vi "Scan stderr.vi"(8 "error in (no error)":errorcluster, 9 "stderr in":u8[](array[numeric]), 10 "patterns":T1, 11 "client in":refnum<class "Generic Client.lvclass">) -> (0 "error out":errorcluster, 1 "stderr out":u8[](array[numeric]), 3 "client out":refnum<class "Generic Client.lvclass">)   [LabVIEW 2020, in "NI_SSH.lvlib" / "Generic Client.lvclass"]
uses:
  <vilib>/net/SSH/Client/Generic/Generic Client.lvclass
  <vilib>/net/SSH/Client/Generic/Stderr Match Patterns.ctl
  <vilib>/net/SSH/Client/Generic/Generic Client.lvclass/Generic Client.ctl
  <vilib>/net/SSH/Client/Generic/Write untrusted fingerprint.vi
  <vilib>/net/SSH/Client/Generic/Write untrusted fingerprint is incorrect_.vi
  <vilib>/Utility/error.llb/Error Cluster From Error Code.vi
  <vilib>/regexp/Match Regular Expression.xnode
  <vilib>/ErrorRing/Error Ring.xnode
  <vilib>/net/SSH/NI_SSH.lvlib
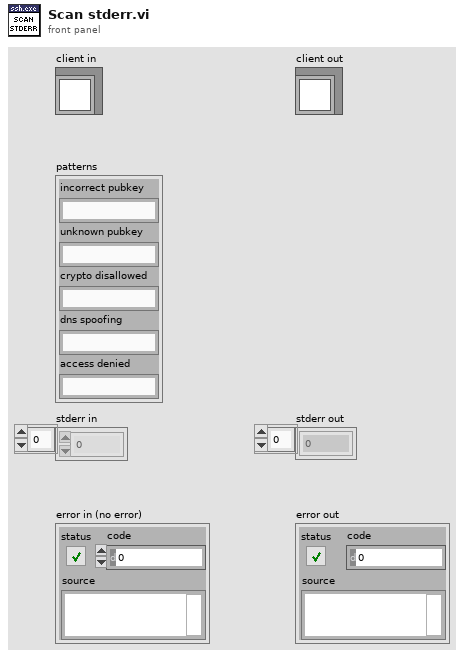
[diagram p1: front panel]
types:
  T1 = typedef "NI_SSH.lvlib/Generic Client.lvclass/Stderr Match Patterns.ctl" = cluster{"incorrect pubkey":string, "unknown pubkey":string, "crypto disallowed":string, "dns spoofing":string, "access denied":string}
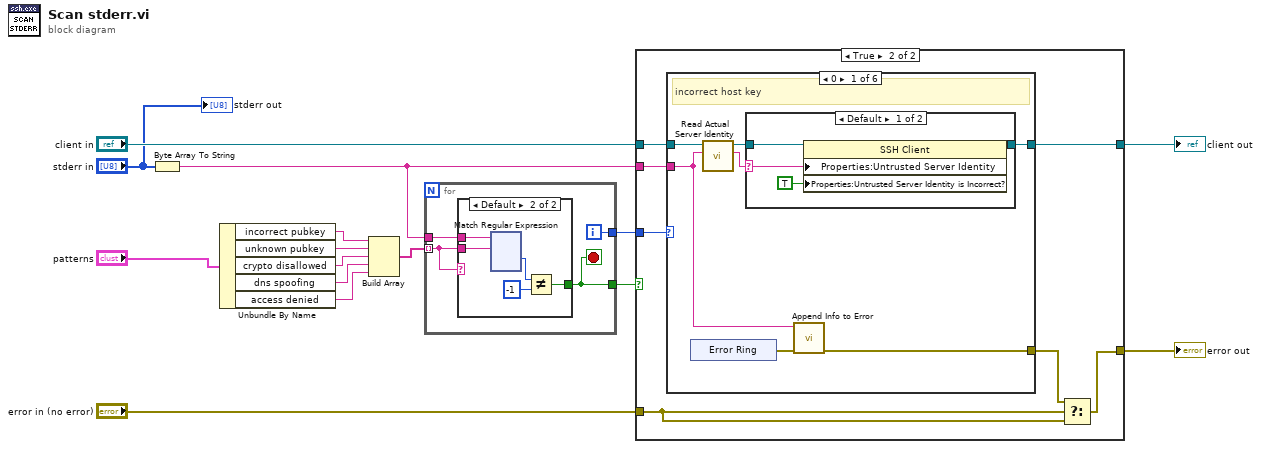
[diagram p0: block diagram]
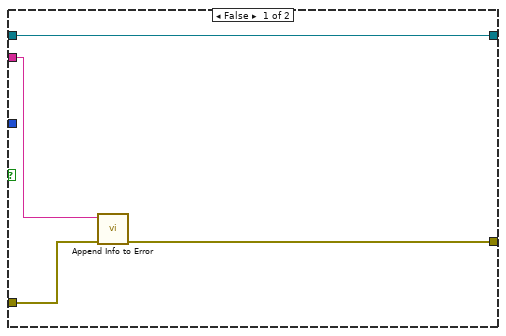
[diagram p2: hidden frame]
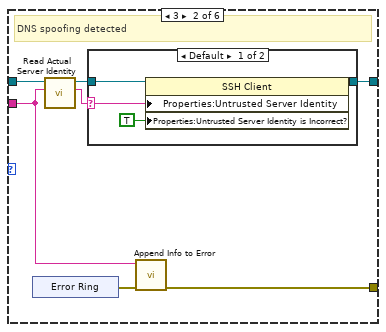
[diagram p4: hidden frame]
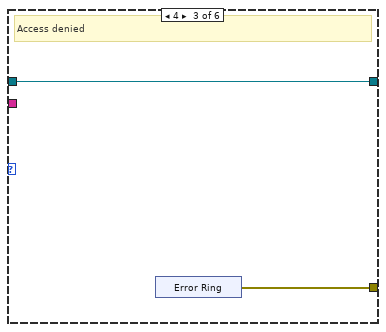
[diagram p6: hidden frame]
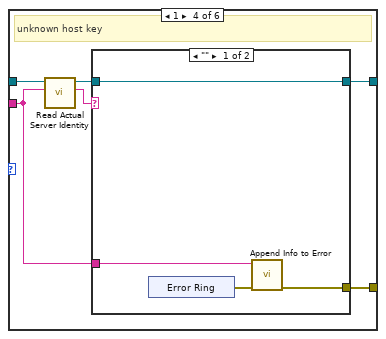
[diagram p7: hidden frame]
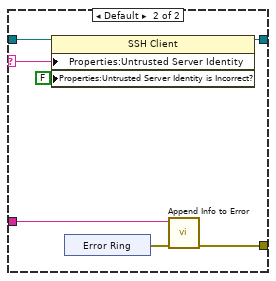
[diagram p8: hidden frame]
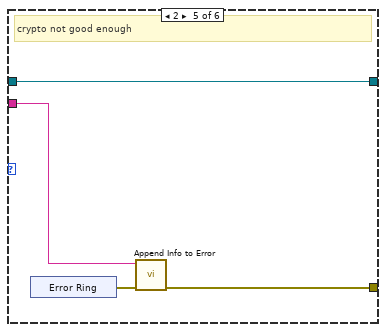
[diagram p9: hidden frame]
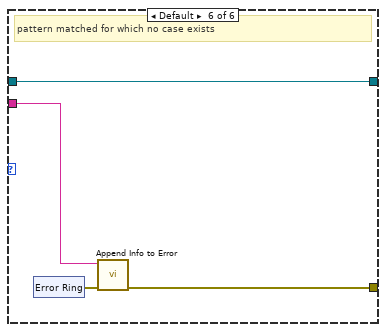
[diagram p10: hidden frame]
diagram:
  n1 = Byte Array To String(unsigned byte array="stderr in") -> (string=w12:string)
  n2 = Unbundle By Name("patterns") -> ("incorrect pubkey"=w6:string, "unknown pubkey"=w5:string, "crypto disallowed"=w4:string, "dns spoofing"=w2:string, "access denied"=w1:string)
  n3 = Build Array(w6, w5, w4, w2, w1) -> (w3:string[])
  n4 = for {
    tunnel: w12 -> [w17]
    tunnel: [w19] -> w8
    tunnel: w3 -> [w16] mode=indexing
    tunnel: [w18] -> w7
    i -> [w18]
    stop <- w19 stop-if-true
    n5 = case shown="Default" w16 {
      tunnel: [_ w23] -> w19
      tunnel: w17 -> [_ w22]
      tunnel: w16 -> [_ w21]
      frame "" {
      }
      frame Default {
        n6 = xnode ("Match Regular Expression")("input string"=w22, "regular expression"=w21) -> ("offset past match"=w20:i32)  [unwired: 4 in, 4 out]
        n7 = Not Equal?(x=w20, y=-1 ("offset past match")) -> (x != y?=w23:bool)
      }
    }
  }
  n8 = case shown="True" w8 {
    tunnel: [w140 w143] -> w11
    tunnel: "error in (no error)" -> [w141 w145]
    tunnel: w12 -> [w139 w148]
    tunnel: "client in" -> [w142 w147]
    tunnel: w7 -> [_ w149]
    tunnel: [w142 w146] -> w15
    frame False {
      n9 = call <vilib>:"Append Info to Error.vi"("error in (no error)"=w141, "additional info"=w139) -> ("error out"=w140:errorcluster)  [unwired: 9 in]
    }
    frame True {
      n10 = case shown="0" w149 {
        tunnel: [w154 w170 w182 w190 w215 w223] -> w144
        tunnel: w148 -> [w152 w168 _ w191 w213 w222]
        tunnel: w147 -> [w150 w166 w183 w188 w216 w224]
        tunnel: [w155 w171 w183 w192 w216 w224] -> w146
        frame 0 {
          # "incorrect host key"
          n11 = xnode ("Error Ring")() -> ("error out"=w153:errorcluster)
          n12 = call-dynamic "Read Actual Server Identity.vi"("server errors"=w152, "client in"=w150) -> ("fingerprint"=w156:string, "client out"=w151:refnum<class "Generic Client.lvclass">)  [unwired: 8 in]
          n13 = case shown="Default" w156 {
            selector: w156 -> [w163 _]
            tunnel: w151 -> [w164 w165]
            tunnel: [w161 w165] -> w155
            frame Default {
              n14 = property on="Property Node" class="SSH Client"(reference=w164, "Properties:Untrusted Server Identity"=w163, "Properties:Untrusted Server Identity is Incorrect?"=TRUE ("untrusted fingerprint is incorrect?")) -> (reference out=w161:refnum<class "Generic Client.lvclass">)  [unwired: 1 in, 1 out]
            }
            frame "" {
            }
          }
          n15 = call <vilib>:"Append Info to Error.vi"("error in (no error)"=w153, "additional info"=w152) -> ("error out"=w154:errorcluster)  [unwired: 9 in]
        }
        frame 3 {
          # "DNS spoofing detected"
          n16 = xnode ("Error Ring")() -> ("error out"=w169:errorcluster)
          n17 = call-dynamic "Read Actual Server Identity.vi"("server errors"=w168, "client in"=w166) -> ("fingerprint"=w172:string, "client out"=w167:refnum<class "Generic Client.lvclass">)  [unwired: 8 in]
          n18 = case shown="Default" w172 {
            selector: w172 -> [w179 _]
            tunnel: w167 -> [w180 w181]
            tunnel: [w177 w181] -> w171
            frame Default {
              n19 = property on="Property Node" class="SSH Client"(reference=w180, "Properties:Untrusted Server Identity"=w179, "Properties:Untrusted Server Identity is Incorrect?"=TRUE ("untrusted fingerprint is incorrect?")) -> (reference out=w177:refnum<class "Generic Client.lvclass">)  [unwired: 1 in, 1 out]
            }
            frame "" {
            }
          }
          n20 = call <vilib>:"Append Info to Error.vi"("error in (no error)"=w169, "additional info"=w168) -> ("error out"=w170:errorcluster)  [unwired: 9 in]
        }
        frame 4 {
          # "Access denied"
          n21 = xnode ("Error Ring")() -> ("error out"=w182:errorcluster)
        }
        frame 1 {
          # "unknown host key"
          n22 = call-dynamic "Read Actual Server Identity.vi"("server errors"=w191, "client in"=w188) -> ("fingerprint"=w193:string, "client out"=w189:refnum<class "Generic Client.lvclass">)  [unwired: 8 in]
          n23 = case shown="\"\"" w193 {
            selector: w193 -> [_ w203]
            tunnel: w189 -> [w197 w205]
            tunnel: [w197 w204] -> w192
            tunnel: w191 -> [w194 w206]
            tunnel: [w196 w208] -> w190
            frame "" {
              n24 = xnode ("Error Ring")() -> ("error out"=w195:errorcluster)
              n25 = call <vilib>:"Append Info to Error.vi"("error in (no error)"=w195, "additional info"=w194) -> ("error out"=w196:errorcluster)  [unwired: 9 in]
            }
            frame Default {
              n26 = property on="Property Node" class="SSH Client"(reference=w205, "Properties:Untrusted Server Identity"=w203, "Properties:Untrusted Server Identity is Incorrect?"=FALSE ("Untrusted Fingerprint is Incorrect?")) -> (reference out=w204:refnum<class "Generic Client.lvclass">)  [unwired: 1 in, 1 out]
              n27 = xnode ("Error Ring")() -> ("error out"=w207:errorcluster)
              n28 = call <vilib>:"Append Info to Error.vi"("error in (no error)"=w207, "additional info"=w206) -> ("error out"=w208:errorcluster)  [unwired: 9 in]
            }
          }
        }
        frame 2 {
          # "crypto not good enough"
          n29 = xnode ("Error Ring")() -> ("error out"=w214:errorcluster)
          n30 = call <vilib>:"Append Info to Error.vi"("error in (no error)"=w214, "additional info"=w213) -> ("error out"=w215:errorcluster)  [unwired: 9 in]
        }
        frame Default {
          # "pattern matched for which no case exists"
          n31 = xnode ("Error Ring")() -> ("error out"=w221:errorcluster)
          n32 = call <vilib>:"Append Info to Error.vi"("error in (no error)"=w221, "additional info"=w222) -> ("error out"=w223:errorcluster)  [unwired: 9 in]
        }
      }
      n33 = Select(t=w144, s=w145, f=w145) -> (s? t:f=w143:errorcluster)
    }
  }
  "client out" <- w15
  "error out" <- w11
  "stderr out" <- "stderr in"
